vi "Protons acceleration inside modules.vi"(2 "Voltage":dbl, 10 "Acceleration":dbl, 11 "Animation in":i32) -> (3 "Accelerated/no":dbl)   [LabVIEW 2020]
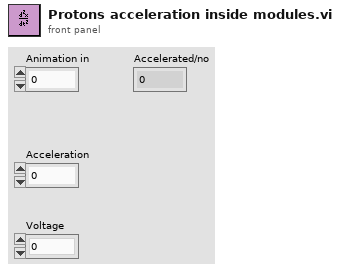
[diagram p1: front panel]
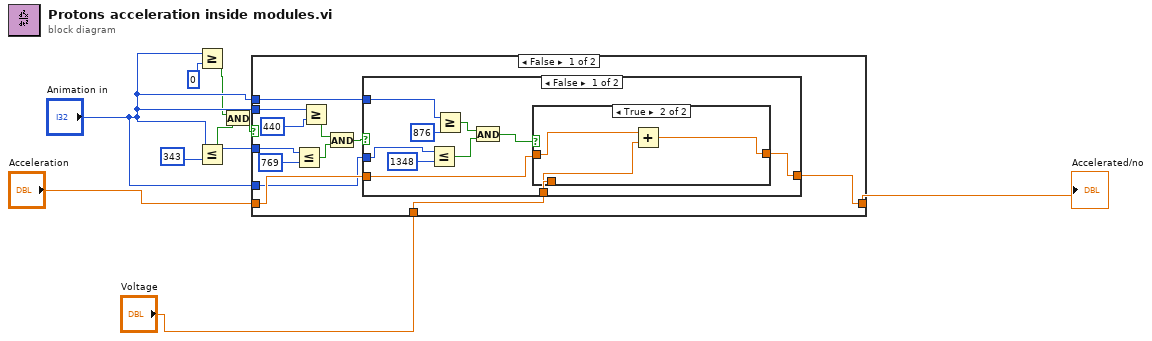
[diagram p0: block diagram]
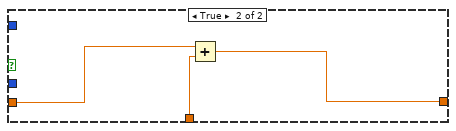
[diagram p3: hidden frame]
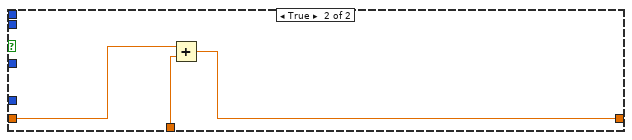
[diagram p4: hidden frame]
diagram:
  n1 = Greater Or Equal?(x="Animation in", y=0) -> (x >= y?=w5:bool)
  n2 = Less Or Equal?(x="Animation in", y=343) -> (x <= y?=w3:bool)
  n3 = And(x=w5, y=w3) -> (x .and. y?=w6:bool)
  n4 = case shown="False" w6 {
    tunnel: "Acceleration" -> [w15 w41]
    tunnel: [w14 w40] -> w8
    tunnel: "Animation in" -> [w13 _]
    tunnel: "Animation in" -> [w17 _]
    tunnel: "Animation in" -> [w12 _]
    tunnel: "Animation in" -> [w11 _]
    tunnel: "Voltage" -> [w10 w39]
    frame False {
      n5 = Less Or Equal?(x=w17, y=769) -> (x <= y?=w19:bool)
      n6 = Greater Or Equal?(x=w13, y=440) -> (x >= y?=w21:bool)
      n7 = And(x=w21, y=w19) -> (x .and. y?=w16:bool)
      n8 = case shown="False" w16 {
        tunnel: w15 -> [w24 w38]
        tunnel: [w23 w37] -> w14
        tunnel: w12 -> [w26 _]
        tunnel: w11 -> [w25 _]
        tunnel: w10 -> [w22 w36]
        frame False {
          n9 = Less Or Equal?(x=w25, y=1348) -> (x <= y?=w30:bool)
          n10 = Greater Or Equal?(x=w26, y=876) -> (x >= y?=w31:bool)
          n11 = And(x=w31, y=w30) -> (x .and. y?=w27:bool)
          n12 = case shown="True" w27 {
            tunnel: w24 -> [w32 w35]
            tunnel: [w32 w34] -> w23
            tunnel: w22 -> [_ w33]
            frame False {
            }
            frame True {
              n13 = Add(x=w35, y=w33) -> (x+y=w34:dbl)
            }
          }
        }
        frame True {
          n14 = Add(x=w38, y=w36) -> (x+y=w37:dbl)
        }
      }
    }
    frame True {
      n15 = Add(x=w41, y=w39) -> (x+y=w40:dbl)
    }
  }
  "Accelerated/no" <- w8
